vi "RichToFlatnidevice_grpc_UnreserveRequest.vi"(5 "OutputClusterType":T1, 11 "InputCluster":T2) -> (3 "OutputCluster":T1)   [LabVIEW 2021, in "NI DAQmx_server.lvlib"]
uses:
  NI DAQmx_server.lvlib
  nidevice_grpc_UnreserveRequest.ctl
  nidevice_grpc_UnreserveRequest_Flat.ctl
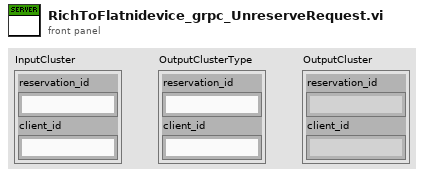
[diagram p1: front panel]
types:
  T1 = typedef "NI DAQmx_server.lvlib/nidevice_grpc_UnreserveRequest_Flat.ctl" = cluster{"reservation_id":string, "client_id":string}
  T2 = typedef "NI DAQmx_server.lvlib/nidevice_grpc_UnreserveRequest.ctl" = cluster{"reservation_id":string, "client_id":string}
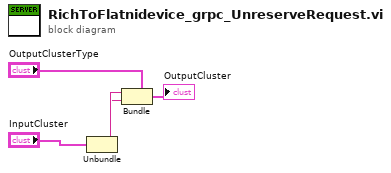
[diagram p0: block diagram]
diagram:
  n1 = Unbundle "Unbundle"("InputCluster") -> ("reservation_id"=w2:string, "client_id"=w1:string)
  n2 = Bundle "Bundle"(cluster="OutputClusterType", "reservation_id"=w2, "client_id"=w1) -> (→"OutputCluster":T1)
